vi "Ready Status.vi"(3 "error in (no error)":errorcluster) -> (1 "error out":errorcluster)   [LabVIEW 2020]
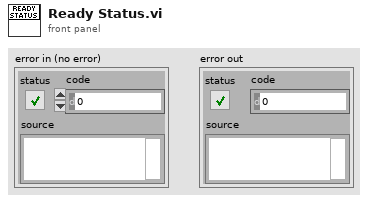
[diagram p1: front panel]
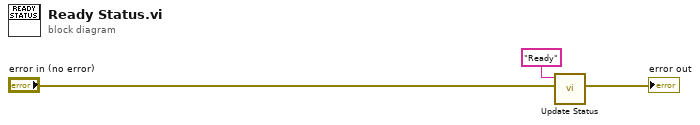
[diagram p0: block diagram]
diagram:
  n1 = call "Update Status.vi"("error in (no error)"="error in (no error)", "Status Bar Text"="Ready") -> ("error out"=→"error out":errorcluster)  [unwired: 9 in]
